vi "StartAcquisition.vi"(8 "error in (no error)":errorcluster, 11 "NIScope in":refnum<class "NIScope.lvclass">) -> (0 "error out":errorcluster, 3 "NIScope out":refnum<class "NIScope.lvclass">)   [LabVIEW 2018, in "ScopePlugins.lvlib" / "NIScope.lvclass"]
uses:
  NIScope.lvclass
  C:/Users/ico/Documents/Projects/NistPluggableModules/Scope/ScopePlugins/ScopePluginBaseClass/ScopePluginsBase.lvclass
  ScopePluginBaseClass/ScopePluginsBase.lvclass/ScopePluginsBase.ctl
  NIScope.lvclass/NIScope.ctl
  ScopePluginBaseClass/Accessors/Read Sync.vi
  Accessors/Read sessions.vi
  ScopePluginBaseClass/Accessors/Read Channels.vi
  Accessors/Write sessions.vi
  <vilib>/Utility/error.llb/Error Cluster From Error Code.vi
  <instrlib>/niSync/niSync.llb/niSync Read Trigger Time Stamp (Single).vi
  <instrlib>/niScope/Acquire/Fetch/niScope Multi Fetch Cluster.vi
  <vilib>/ErrorRing/Error Ring.xnode
panel:
  out "RelativeInitialX":dbl[](array[numeric])
  out "AbsTimeOffset":timestamp[](array[timestamp])
  out "trigger time":timestamp
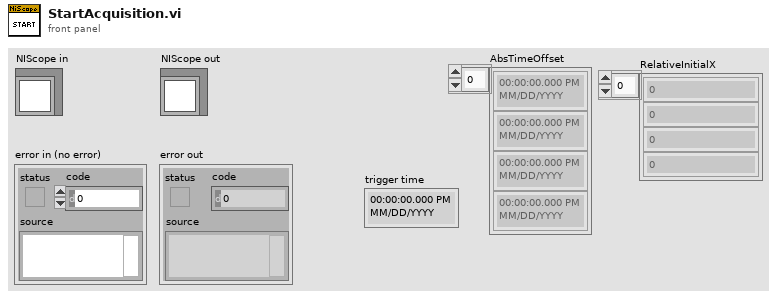
[diagram p1: front panel]
types:
  T1 = typedef "ScopePlugins.lvlib/Channels.ctl" = cluster{"Count":i32, "ChannelArray":T2[]}
  T2 = typedef "ScopePlugins.lvlib/Channel.ctl" = cluster{"Enabled":bool, "Name":string, "InputImpedance":dbl, "InputFreqMax":dbl, "ProbeAttn":dbl, "Coupling":enum16{"AC", "DC", "GND"}, "Offset":dbl, "Range":dbl, "Handle":string, "Connected":bool, "Options String ":string}
  T3 = typedef "ScopePlugins.lvlib/ScopePluginsBase.lvclass/Sync.ctl" = cluster{"Handle":string, "SrcTerm":string, "DestTerm":string}
  T4 = cluster{"instrument handle":refnum<k15>, string}[]
  T5 = cluster{"relativeInitialX":dbl, "xIncrement":dbl, "wfm":dbl[]}[]
  T6 = cluster{"actualSamples":i32, "absoluteInitialX":dbl, "relativeInitialX":dbl, "xIncrement":dbl, "offset":dbl, "gain":dbl, "reserved1":dbl, "reserved2":dbl}[]
  T7 = cluster{"relativeInitialX":dbl, "xIncrement":dbl, "wfm":dbl[]}
  T8 = cluster{"actualSamples":i32, "absoluteInitialX":dbl, "relativeInitialX":dbl, "xIncrement":dbl, "offset":dbl, "gain":dbl, "reserved1":dbl, "reserved2":dbl}
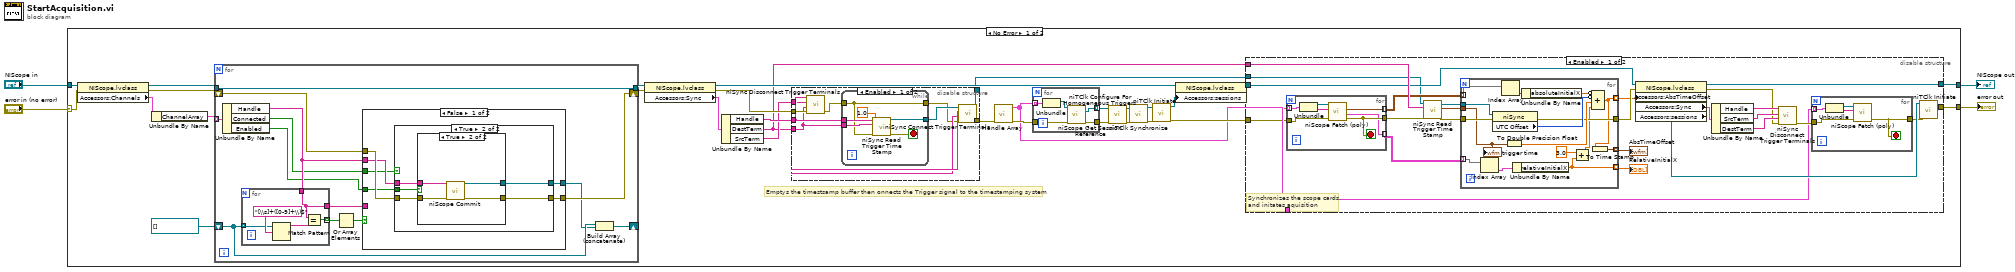
[diagram p0: block diagram]
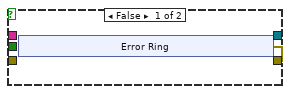
[diagram p4: hidden frame]
diagram:
  n1 = case shown="No Error" "error in (no error)" {
    selector: "error in (no error)" -> [w33 w154]
    tunnel: "NIScope in" -> [w34 w155]
    tunnel: [w23 w155] -> w2
    tunnel: [w18 w154] -> w1
    frame No Error {
      # "Emptys the timestsamp buffer then onnects the Trigger signal to the timestamping system"
      n2 = property class="NIScope.lvclass"(reference=w34, error in=w33) -> (reference out=w30:refnum<class "NIScope.lvclass">, error out=w28:errorcluster, "Accessors:Channels"=w32:T1)
      n3 = Unbundle By Name(w32) -> ("ChannelArray"=w29:T2[])
      n4 = for {
        tunnel: w29 -> [w123] mode=indexing
        shift-right: [w118] -> w26
        shift-left: w28 -> [w119]
        shift-right: [w120] -> _
        shift-left: refnum<k15>[] [] -> [w121]
        tunnel: w30 -> [w117]
        tunnel: [w117] -> w27
        n5 = Unbundle By Name(w123) -> ("Handle"=w116:string, "Connected"=w112:bool, "Enabled"=w111:bool)
        n6 = for {
          tunnel: w121 -> [w150] mode=indexing
          tunnel: w116 -> [w151]
          tunnel: [w151] -> w122
          tunnel: [w149] -> w114 mode=indexing
          n7 = Match Pattern(string=w150, regular expression="[\\s]+([0-9]+\\)$") -> (before substring=w152:string)  [unwired: 1 in, 3 out]
          n8 = Equal?(x=w151, y=w152) -> (x = y?=w149:bool)
        }
        n9 = Or Array Elements(Boolean array=w114) -> (logical OR=w113:bool)
        n10 = case shown="False" w113 {
          tunnel: w122 -> [_ w147]
          tunnel: [w129 w148] -> w118
          tunnel: [w128 w147] -> w115
          tunnel: w119 -> [w127 w148]
          tunnel: w116 -> [w126 _]
          tunnel: w112 -> [w125 _]
          tunnel: w111 -> [w124 _]
          frame False {
            n11 = case shown="True" w125 {
              tunnel: [w130 w140] -> w129
              tunnel: [_ w139] -> w128
              tunnel: w127 -> [_ w138]
              tunnel: w126 -> [_ w137]
              tunnel: w124 -> [_ w136]
              frame False {
                n12 = xnode "Error Ring"() -> ("error out"=w130:errorcluster)
              }
              frame True {
                n13 = case shown="True" w136 {
                  tunnel: [w141 w143] -> w140
                  tunnel: [w142 w144] -> w139
                  tunnel: w138 -> [w141 w145]
                  tunnel: w137 -> [w142 w146]
                  frame False {
                  }
                  frame True {
                    n14 = call <instrlib>:"niScope Commit.vi"("instrument handle"=w146, "error in"=w145) -> ("instrument handle out"=w144:refnum<k15>, "error out"=w143:errorcluster)  [unwired: 12 in]
                  }
                }
              }
            }
          }
          frame True {
          }
        }
        n15 = Build Array (concatenate)(w121, w115) -> (w120:refnum<k15>[])
      }
      n16 = property class="NIScope.lvclass"(reference=w27, error in=w26) -> (reference out=w24:refnum<class "NIScope.lvclass">, error out=w22:errorcluster, "Accessors:Sync"=w25:T3)
      n17 = Unbundle By Name(w25) -> ("Handle"=w21:string, "DestTerm"=w19:string, "SrcTerm"=w20:string)
      n18 = disable-structure shown="Enabled" {
        disable-tunnel: w22 -> [w98 w105]
        disable-tunnel: w21 -> [w97 _]
        disable-tunnel: w20 -> [w96 _]
        disable-tunnel: w19 -> [w95 _]
        disable-tunnel: [w93 _] -> w12
        disable-tunnel: [w90 w105] -> w5
        frame Enabled {
          n19 = call <instrlib>:"niSync Disconnect Trigger Terminals.vi"("error in (no error)"=w98, "destination terminal"=w95, "source terminal"=w96, "instrument handle"=w97) -> ("error out"=w94:errorcluster)  [unwired: 6 in, 1 out]
          n20 = while {
            tunnel: w97 -> [w104]
            tunnel: w95 -> [w103]
            tunnel: [w100] -> w92
            tunnel: w94 -> [w99]
            tunnel: [w99] -> w91
            stop <- w101 stop-if-true
            n21 = call-poly <instrlib>:"niSync Read Trigger Time Stamp.vi"("instrument handle"=w104, "terminal"=w103, "timeout"=1.0, "error in (no error)"=w99) -> ("instrument handle out"=w100:refnum<k15>, "error out"=w101:errorcluster)  [unwired: 8 in, 2 out]
          }
          n22 = call <instrlib>:"niSync Connect Trigger Terminals.vi"("error in (no error)"=w91, "destination terminal"=w95, "source terminal"=w96, "instrument handle"=w92) -> ("error out"=w90:errorcluster, "instrument handle out"=w93:refnum<k15>)  [unwired: 6 in]
        }
        frame Disabled {
        }
      }
      n23 = call "Handle Array.vi"("error in (no error)"=w5) -> ("error out"=w10:errorcluster, "Array Handles"=w6:T4)  [unwired: 9 in]
      n24 = for {
        tunnel: w10 -> [w110]
        tunnel: [w109] -> w9
        tunnel: [w108] -> w7 mode=indexing
        tunnel: w6 -> [w107] mode=indexing
        n25 = Unbundle(w107) -> ("instrument handle"=w106:refnum<k15>)  [unwired: 1 out]
        n26 = call <instrlib>:"niScope Get Session Reference.vi"("instrument handle"=w106, "error in"=w110) -> ("session reference"=w108:refnum<k20>, "error out"=w109:errorcluster)  [unwired: 11 in, 1 out]
      }
      n27 = call <instrlib>:"niTClk Configure For Homogeneous Triggers.vi"("error in (no error)"=w9, "sessions"=w7) -> ("error out"=w14:errorcluster, "sessions out"=w17:refnum<k20>[])  [unwired: 8 in]
      n28 = call <instrlib>:"niTClk Synchronize.vi"("error in (no error)"=w14, "sessions"=w17) -> ("error out"=w11:errorcluster, "sessions out"=w16:refnum<k20>[])  [unwired: 8 in]
      n29 = call <instrlib>:"niTClk Initiate.vi"("error in (no error)"=w11, "sessions"=w16) -> ("error out"=w8:errorcluster, "sessions out"=w15:refnum<k20>[])  [unwired: 8 in]
      n30 = property class="NIScope.lvclass"(reference=w24, "Accessors:sessions"=w15) -> (reference out=w13:refnum<class "NIScope.lvclass">)  [unwired: 1 in, 1 out]
      n31 = disable-structure shown="Enabled" {
        disable-tunnel: [w59 w89] -> w23
        disable-tunnel: w19 -> [w58 _]
        disable-tunnel: [w57 w88] -> w18
        disable-tunnel: w13 -> [w51 w89]
        disable-tunnel: w12 -> [w37 _]
        disable-tunnel: w8 -> [w36 w88]
        disable-tunnel: w6 -> [w35 _]
        frame Enabled {
          # "Synchronizes the scope cards\nand initates aquisition"
          n32 = for {
            tunnel: w36 -> [w84]
            tunnel: w35 -> [w87] mode=indexing
            tunnel: [w83] -> w55 mode=indexing
            tunnel: [w82] -> w56
            tunnel: [w81] -> w39 mode=indexing
            stop <- w82 stop-if-true
            n33 = Unbundle(w87) -> ("instrument handle"=w85:refnum<k15>, w86:string)
            n34 = call-poly <instrlib>:"niScope Fetch (poly).vi"("error in"=w84, "channels"=w86, "instrument handle"=w85) -> ("error out"=w82:errorcluster, "waveform"=w81:T5, "wfm info"=w83:T6)  [unwired: 5 in, 1 out]
          }
          n35 = call-poly <instrlib>:"niSync Read Trigger Time Stamp.vi"("instrument handle"=w37, "terminal"=w58, "error in (no error)"=w56) -> ("instrument handle out"=w54:refnum<k15>, "time stamp out"=w53:timestamp, "error out"=w52:errorcluster)  [unwired: 9 in, 1 out]
          n36 = for {
            tunnel: w55 -> [w80] mode=indexing
            tunnel: w54 -> [w78]
            tunnel: w53 -> [w76]
            tunnel: w52 -> [w77]
            tunnel: [w70] -> w49 mode=indexing
            tunnel: [w72] -> w50
            tunnel: [w71] -> w43 mode=indexing
            tunnel: w39 -> [w69] mode=indexing
            tunnel: [w67] -> w38 mode=indexing
            n37 = Index Array(array=w69) -> (element=w68:T7)  [unwired: 1 in]
            n38 = property class="niSync"(reference=w78, error in=w77) -> (error out=w72:errorcluster, "UTC Offset"=w74:i32)  [unwired: 1 out]
            n39 = Index Array(array=w80) -> (element=w79:T8)  [unwired: 1 in]
            n40 = To Double Precision Float(number=w76) -> (double precision float=w73:dbl)
            n41 = Unbundle By Name(w68) -> ("relativeInitialX"=w67:dbl)
            n42 = Unbundle By Name(w79) -> ("absoluteInitialX"=w75:dbl)
            n43 = Add(x=3.0, y=w67) -> (x+y=w66:dbl)
            n44 = Compound Arithmetic op=ADD(invert w75, invert w74, w73, w66) -> (w70:dbl)
            n45 = To Time Stamp(1:w70) -> (0:w71:timestamp)
            "trigger time" <- w76
          }
          "AbsTimeOffset" <- w43
          "RelativeInitialX" <- w38
          n46 = property class="NIScope.lvclass"(reference=w51, error in=w50, "Accessors:AbsTimeOffset"=w49) -> (reference out=w59:refnum<class "NIScope.lvclass">, error out=w44:errorcluster, "Accessors:Sync"=w48:T3, "Accessors:sessions"=w42:refnum<k20>[])
          n47 = Unbundle By Name(w48) -> ("Handle"=w47:string, "SrcTerm"=w46:string, "DestTerm"=w45:string)
          n48 = call <instrlib>:"niSync Disconnect Trigger Terminals.vi"("error in (no error)"=w44, "destination terminal"=w45, "source terminal"=w46, "instrument handle"=w47) -> ("error out"=w41:errorcluster)  [unwired: 6 in, 1 out]
          n49 = for {
            tunnel: w41 -> [w61]
            tunnel: w35 -> [w64] mode=indexing
            tunnel: [w60] -> w40
            stop <- w60 stop-if-true
            n50 = Unbundle(w64) -> ("instrument handle"=w62:refnum<k15>, w63:string)
            n51 = call-poly <instrlib>:"niScope Fetch (poly).vi"("error in"=w61, "channels"=w63, "instrument handle"=w62) -> ("error out"=w60:errorcluster)  [unwired: 5 in, 3 out]
          }
          n52 = call <instrlib>:"niTClk Initiate.vi"("error in (no error)"=w40, "sessions"=w42) -> ("error out"=w57:errorcluster)  [unwired: 8 in, 1 out]
        }
        frame Disabled {
        }
      }
    }
    frame Error {
    }
  }
  "error out" <- w1
  "NIScope out" <- w2
